vi "TL hindbrain ACT.vi"(0 "Manual\nRudder":dbl min=-45.0 max=45.0 step=1.0, 1 "Manual\nSpeed":dbl min=-9.0 max=9.0 step=1.0, 2 "Act Com":T1, 3 "error in":errorcluster, 4 "Manual?":bool) -> (5 "Rudder":dbl min=-45.0 max=45.0 step=1.0, 6 "Speed":dbl min=-9.0 max=9.0 step=1.0, 7 "error out":errorcluster)   [LabVIEW 2014]
doc: "This vi has two functions: it selects between manual and auto mode and it converts the incoming value into speed and rudder control values."
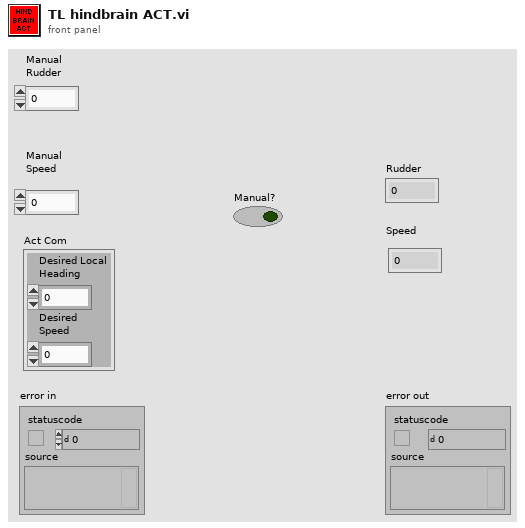
[diagram p1: front panel]
types:
  T1 = cluster{"Desired Local\nHeading":dbl, "Desired\nSpeed":dbl}
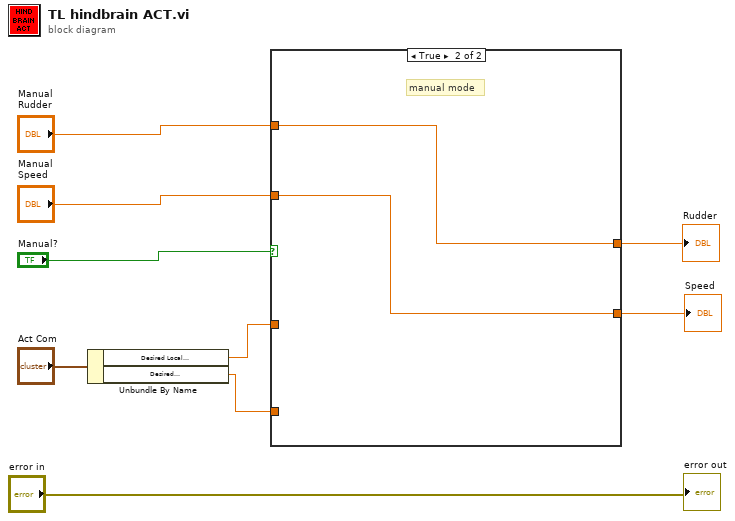
[diagram p0: block diagram]
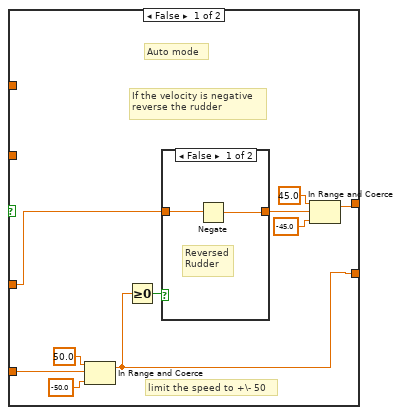
[diagram p2: hidden frame]
diagram:
  n1 = Unbundle By Name("Act Com") -> ("Desired Local\nHeading"=w2:dbl, "Desired\nSpeed"=w3:dbl)
  n2 = case shown="True" "Manual?" {
    tunnel: [w15 w24] -> w8
    tunnel: [w13 w23] -> w7
    tunnel: "Manual\nRudder" -> [_ w24]
    tunnel: "Manual\nSpeed" -> [_ w23]
    tunnel: w3 -> [w14 _]
    tunnel: w2 -> [w11 _]
    frame False {
      # "If the velocity is negative \nreverse the rudder"
      # "limit the speed to +\\- 50"
      # "Auto mode"
      n3 = In Range and Coerce(upper limit=50.0, x=w14, lower limit=-50.0) -> (coerced(x)=w13:dbl)  [unwired: 1 out]
      n4 = Greater Or Equal To 0?(x=w13) -> (x >= 0?=w12:bool)
      n5 = case shown="False" w12 {
        tunnel: w11 -> [w21 w22]
        tunnel: [w20 w22] -> w10
        frame False {
          # "Reversed\nRudder"
          n6 = Negate(x=w21) -> (-x=w20:dbl)
        }
        frame True {
          # "Normal\nRudder"
        }
      }
      n7 = In Range and Coerce(upper limit=45.0, x=w10, lower limit=-45.0) -> (coerced(x)=w15:dbl)  [unwired: 1 out]
    }
    frame True {
      # "manual mode"
    }
  }
  "Rudder" <- w8
  "Speed" <- w7
  "error out" <- "error in"
